vi "CreateCurveNames.vi"(0 "Exp.lvclass In":refnum<class "Experiment.lvclass">, 5 "IndCourbe":i64 caption="Numéro de Balayage", 7 "SinglePar":bool, 9 "NomDon":string[](array[string])=["RTêta;", "X&Y;"], 11 "error in":errorcluster, 12 "ScanFunc":i32) -> (2 "MultiScan":bool, 3 "ScanTableSize":i32[](array[numeric]), 4 "Experiment.lvclass Out":refnum<class "Experiment.lvclass">, 6 "Scan list":string[](array[string]), 10 "VarPar list":string[](array[string]), 13 "CalcQIndex":cluster{"Tableau":i32[]}[](array[cluster]), 14 "DataQIndex":cluster{"Tableau":i32[]}[](array[cluster]), 15 "error out":errorcluster)   [LabVIEW 2019, in "Experiment.lvclass"]
doc: "Ce Vi créer la ligne d'entête du fichier texte de sauvegarde à partir du nombre de courbe voulu."
uses:
  Experiment.lvclass
  Experiment.lvclass/Experiment.ctl
  Calculations Class/Calculations.lvclass
  Calculations Class/Calculations.lvclass/Calculations.ctl
  Calculations Class/Accessor/GetCalcEveryScanPar.vi
  DevicesClass/BaseDevice/BaseDevice.lvclass
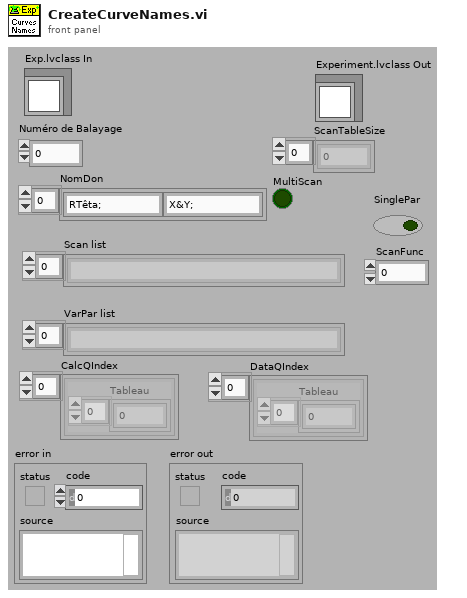
[diagram p1: front panel]
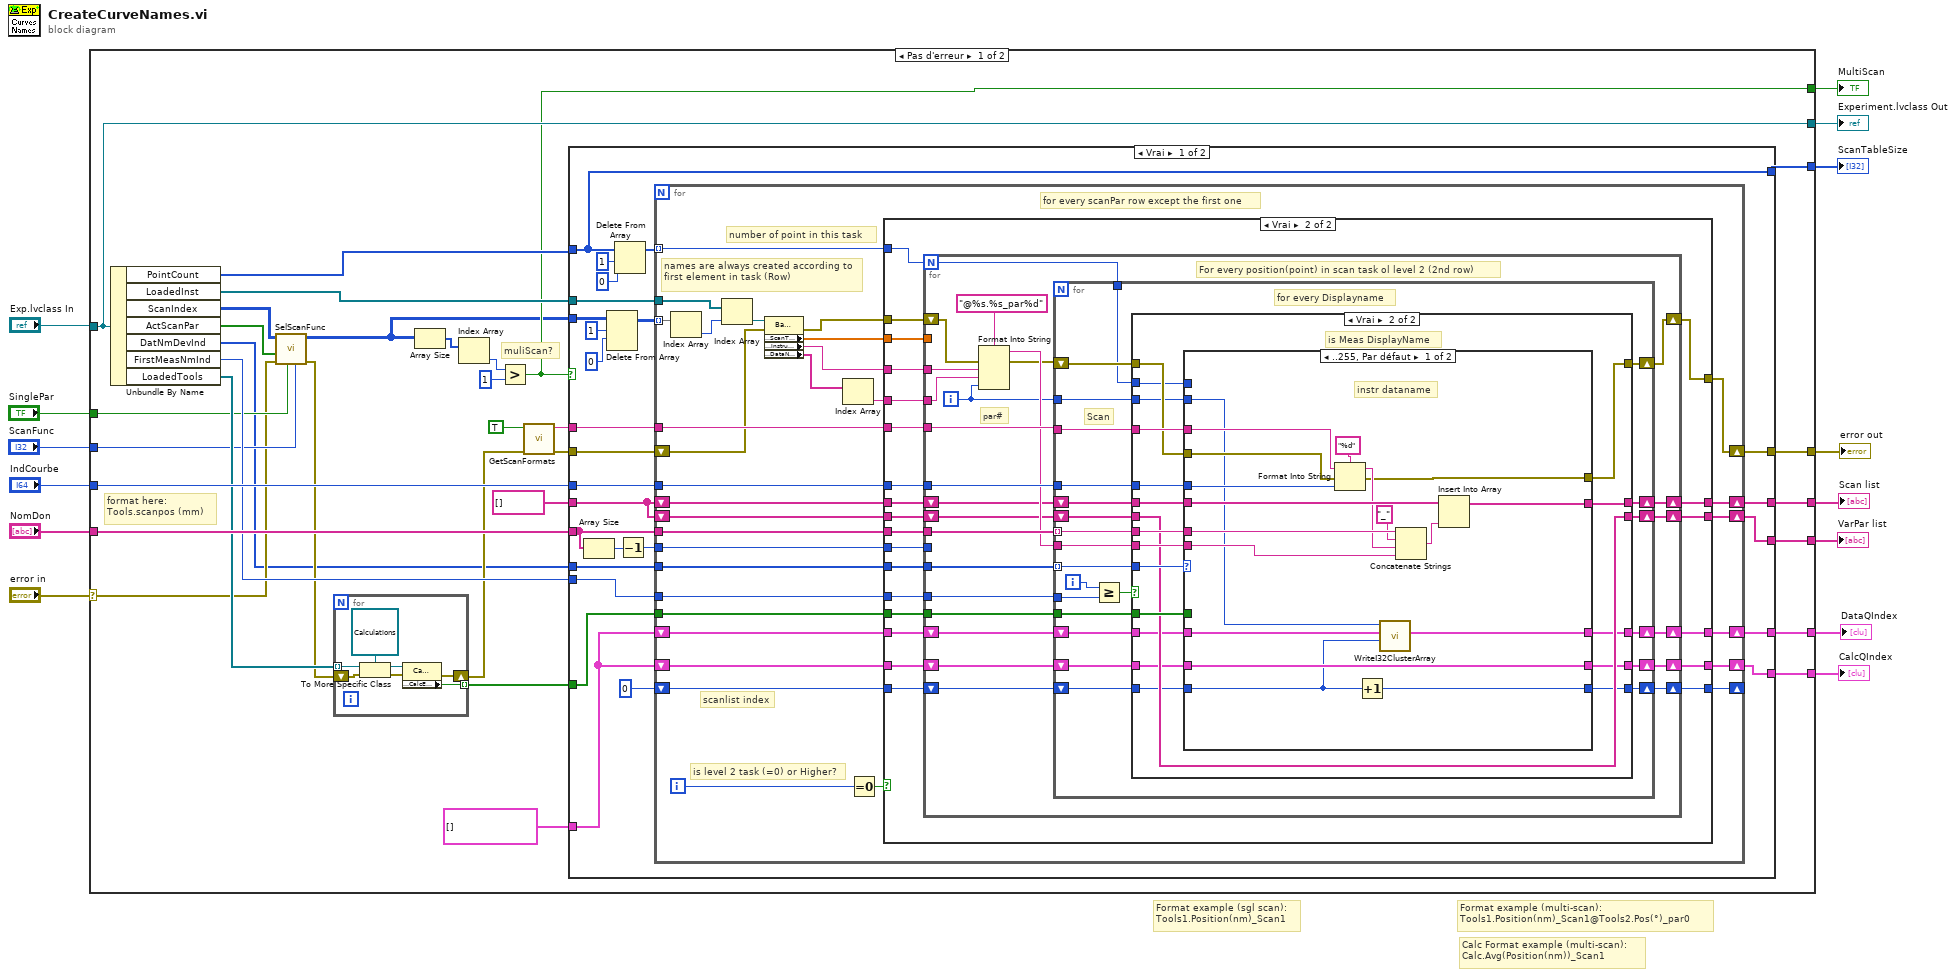
[diagram p0: block diagram]
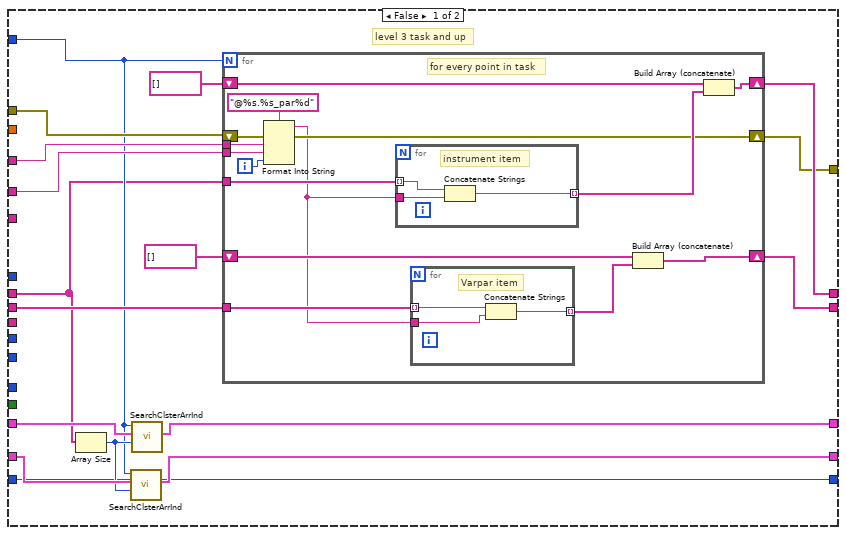
[diagram p2: hidden frame]
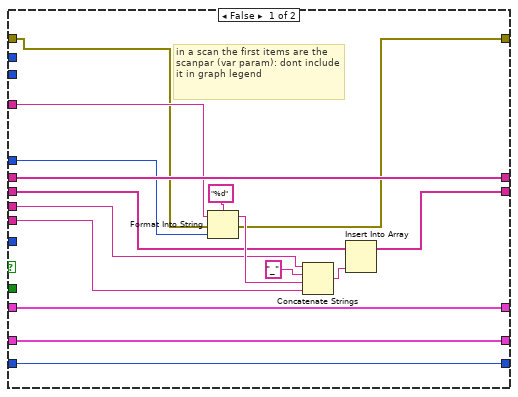
[diagram p3: hidden frame]
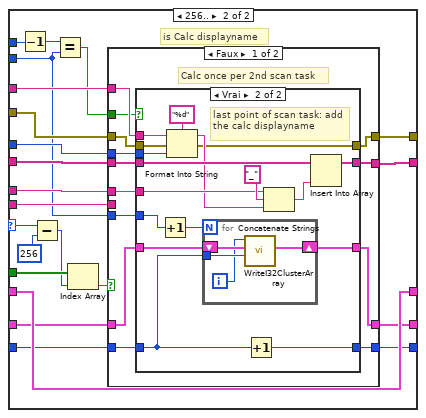
[diagram p4: hidden frame]
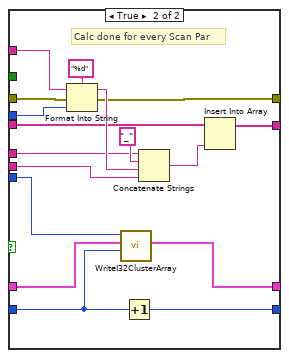
[diagram p6: hidden frame]
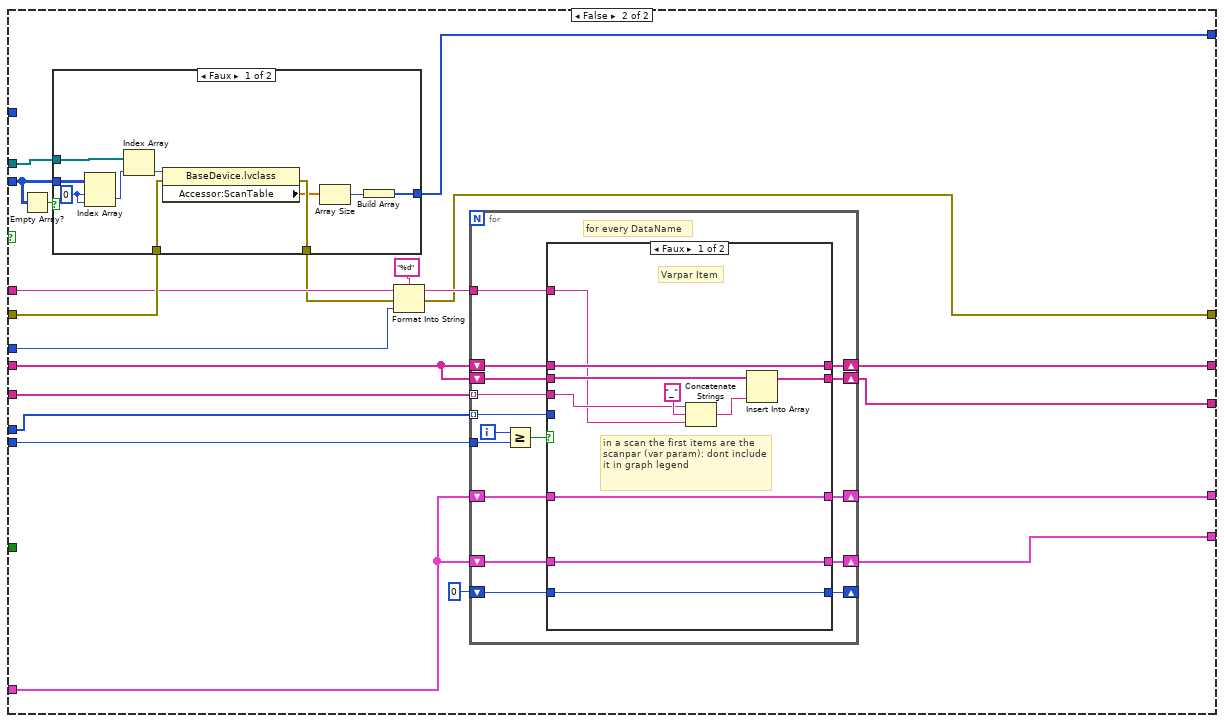
[diagram p7: hidden frame]
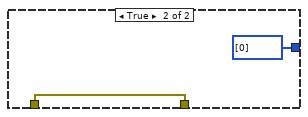
[diagram p8: hidden frame]
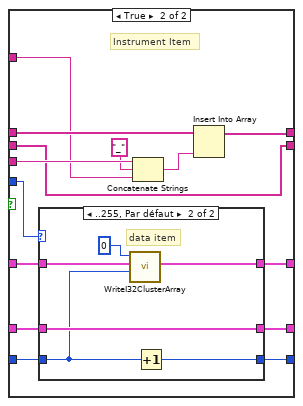
[diagram p9: hidden frame]
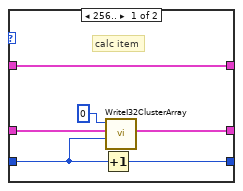
[diagram p10: hidden frame]
diagram:
  # "Calc Format example (multi-scan):\nCalc.Avg(Position(nm))_Scan1"
  # "Format example (multi-scan):\nTools1.Position(nm)_Scan1@Tools2.Pos(°)_par0"
  # "Format example (sgl scan):\nTools1.Position(nm)_Scan1"
  n1 = case shown="Pas d'erreur" "error in" {
    selector: "error in" -> [w18 w436]
    tunnel: [w38 w436] -> w13
    tunnel: [w42 _] -> w12
    tunnel: "NomDon" -> [w43 _]
    tunnel: "Exp.lvclass In" -> [w29 w435]
    tunnel: "IndCourbe" -> [w45 _]
    tunnel: [w29 w435] -> w8
    tunnel: [w36 _] -> w7
    tunnel: [w28 _] -> w6
    tunnel: [w26 _] -> w5
    tunnel: [w25 _] -> w4
    tunnel: "SinglePar" -> [w20 _]
    tunnel: "ScanFunc" -> [w19 _]
    tunnel: [w23 _] -> w1
    frame No Error {
      # "format here:\nTools.scanpos (mm)"
      # "muliScan?"
      n2 = Unbundle By Name(w29) -> ("PointCount"=w33:i32[], "LoadedInst"=w39:refnum<class "BaseDevice.lvclass">[], "ScanIndex"=w22:i32[][], "ActScanPar"=w15:bool[], "DatNmDevInd"=w16:i32[], "FirstMeasNmInd"=w37:i32, "LoadedTools"=w32:refnum<class "BaseDevice.lvclass">[])
      n3 = call "SelScanFunc.vi"("Function"=w19, "SInglePar"=w20, "ErrorIn(No Error)"=w18, "Active ScanPar"=w15, "ScanIndexIn"=w22) -> ("sortie d'erreur"=w17:errorcluster, "ScanIndexOut"=w21:i32[][])  [unwired: 4 in, 1 out]
      n4 = for {
        tunnel: w32 -> [w50] mode=indexing
        shift-right: [w48] -> w31
        shift-left: w17 -> [w49]
        tunnel: [w47] -> w30 mode=indexing
        n5 = To More Specific Class(target class=refnum<class "Calculations.lvclass"> refnum ("Calculations.lvclass"), reference=w50, error in=w49) -> (specific class reference=w52:refnum<class "Calculations.lvclass">, error out=w53:errorcluster)
        n6 = property class="Calculations.lvclass"(reference=w52, error in=w53) -> (error out=w48:errorcluster, "Accessor:CalcEveryScanPar"=w47:bool)  [unwired: 1 out]
      }
      n7 = Array Size(array=w21) -> (size(s)=w35:i32[])
      n8 = Index Array(array=w35) -> (element=w34:i32)  [unwired: 1 in]
      n9 = Greater?(x=w34, y=1) -> (0:w23:bool)
      n10 = call "GetScanFormats.vi"("ErrorIn(No Error)"=w31, "Scan(T)"=TRUE) -> ("sortie d'erreur"=w44:errorcluster, "Prefixe"=w46:string)  [unwired: 7 in, 1 out]
      n11 = case shown="Vrai" w23 {
        tunnel: w46 -> [w79 w360]
        tunnel: w45 -> [w78 w361]
        tunnel: w44 -> [w77 w365]
        tunnel: w43 -> [w64 w370]
        tunnel: [w72 w369] -> w42
        tunnel: string[] [] -> [w59 w364]
        tunnel: w21 -> [w76 w351]
        tunnel: w39 -> [w75 w367]
        tunnel: [w74 w353] -> w38
        tunnel: w37 -> [w73 w368]
        tunnel: [w60 w366] -> w36
        tunnel: w33 -> [w60 _]
        tunnel: w16 -> [w65 w357]
        tunnel: w30 -> [w61 _]
        tunnel: [w58 w363] -> w28
        tunnel: cluster{"Tableau":i32[]}[] [] ("CalcQIndex") -> [w56 w355]
        tunnel: [w55 w354] -> w26
        tunnel: [w54 w356] -> w25
        frame True {
          n12 = Array Size(array=w64) -> (size(s)=w63:i32)
          n13 = Delete From Array(array=w76, length=1 ("longueur"), index (row)=0 ("indice (ligne)")) -> (array with subset deleted=w71:i32[][])  [unwired: 1 in, 1 out]
          n14 = Delete From Array(array=w60, length=1 ("longueur"), index=0 ("indice")) -> (array with subset deleted=w67:i32[])  [unwired: 1 out]
          n15 = Decrement(x=w63) -> (x-1=w62:i32)
          n16 = for {
            tunnel: w79 -> [w110]
            tunnel: w78 -> [w109]
            tunnel: w64 -> [w108]
            tunnel: w71 -> [w107] mode=indexing
            tunnel: w75 -> [w106]
            shift-right: [w104] -> w74
            shift-left: w77 -> [w105]
            tunnel: w73 -> [w103]
            shift-right: [w100] -> w72
            shift-left: w59 -> [w99]
            tunnel: w67 -> [w80] mode=indexing
            tunnel: w65 -> [w92]
            tunnel: w61 -> [w91]
            tunnel: w62 -> [w90]
            shift-right: [w87] -> w58
            shift-left: w59 -> [w88]
            shift-right: [w85] -> _
            shift-left: 0 ("Numérique") -> [w86]
            shift-right: [w81] -> w55
            shift-left: w56 -> [w82]
            shift-right: [w83] -> w54
            shift-left: w56 -> [w84]
            i -> [w89]
            # "scanlist index"
            # "is level 2 task (=0) or Higher?"
            # "number of point in this task"
            # "names are always created according to first element in task (Row)"
            # "for every scanPar row except the first one"
            n17 = Index Array(array=w107) -> (element=w97:i32)  [unwired: 1 in]
            n18 = Index Array(array=w106, index=w97) -> (element=w96:refnum<class "BaseDevice.lvclass">)
            n19 = property class="BaseDevice.lvclass"(reference=w96, error in=w105) -> (error out=w98:errorcluster, "Accessor:ScanTable"=w94:dbl[], "Accessor:InstrumentName"=w101:string, "Accessor:DataNames"=w95:string[])  [unwired: 1 out]
            n20 = Index Array(array=w95) -> (element=w102:string)  [unwired: 1 in]
            n21 = Equal To 0?(x=w89) -> (x = 0?=w93:bool)
            n22 = case shown="Vrai" w93 {
              tunnel: w110 -> [_ w171]
              tunnel: w109 -> [_ w170]
              tunnel: w108 -> [_ w169]
              tunnel: [w125 w168] -> w104
              tunnel: w103 -> [_ w167]
              tunnel: w102 -> [w124 w166]
              tunnel: w101 -> [w123 w165]
              tunnel: [w126 w164] -> w100
              tunnel: w99 -> [w111 w163]
              tunnel: w80 -> [w112 w149]
              tunnel: w98 -> [w127 w162]
              tunnel: w94 -> [_ w161]
              tunnel: w92 -> [_ w160]
              tunnel: w91 -> [_ w159]
              tunnel: w90 -> [_ w158]
              tunnel: w88 -> [w119 w157]
              tunnel: [w122 w156] -> w87
              tunnel: w86 -> [w113 w155]
              tunnel: [w113 w154] -> w85
              tunnel: w84 -> [w118 w153]
              tunnel: [w115 w152] -> w83
              tunnel: w82 -> [w117 w151]
              tunnel: [w114 w150] -> w81
              frame False {
                # "level 3 task and up"
                n23 = Array Size(array=w111) -> (size(s)=w116:i32)
                n24 = call "SearchClsterArrInd.vi"("ScanlistSize"=w116, "array"=w117, "Currtaskparcnt"=w112) -> ("output array"=w114:cluster{"Tableau":i32[]}[])  [unwired: 7 in, 1 out]
                n25 = call "SearchClsterArrInd.vi"("ScanlistSize"=w116, "array"=w118, "Currtaskparcnt"=w112) -> ("output array"=w115:cluster{"Tableau":i32[]}[])  [unwired: 7 in, 1 out]
                n26 = for {
                  N: w112 -> [_]
                  tunnel: w123 -> [w142]
                  tunnel: w124 -> [w141]
                  shift-right: [w137] -> w125
                  shift-left: w127 -> [w140]
                  tunnel: w111 -> [w139]
                  shift-right: [w136] -> w126
                  shift-left: string[] [] -> [w135]
                  shift-right: [w133] -> w122
                  shift-left: string[] [] -> [w132]
                  tunnel: w119 -> [w131]
                  i -> [w128]
                  # "for every point in task"
                  n27 = Format Into String(format string="@%s.%s_par%d" ("chaîne de format"), error in=w140, w142, w141, w128) -> (resulting string=w129:string, error out=w137:errorcluster)  [unwired: 1 in]
                  n28 = for {
                    tunnel: w139 -> [w143] mode=indexing
                    tunnel: [w145] -> w138 mode=indexing
                    tunnel: w129 -> [w144]
                    # "instrument item"
                    n29 = Concatenate Strings(w143, w144) -> (w145:string)
                  }
                  n30 = for {
                    tunnel: w131 -> [w148] mode=indexing
                    tunnel: [w147] -> w134 mode=indexing
                    tunnel: w129 -> [w146]
                    # "Varpar item"
                    n31 = Concatenate Strings(w148, w146) -> (w147:string)
                  }
                  n32 = Build Array (concatenate)(w132, w134) -> (w133:string[])
                  n33 = Build Array (concatenate)(w135, w138) -> (w136:string[])
                }
              }
              frame True {
                n34 = for {
                  N: w149 -> [w183]
                  tunnel: w171 -> [w196]
                  tunnel: w170 -> [w195]
                  tunnel: w169 -> [w194]
                  shift-right: [w180] -> w168
                  shift-left: w162 -> [w192]
                  tunnel: w167 -> [w193]
                  tunnel: w166 -> [w191]
                  tunnel: w165 -> [w190]
                  shift-right: [w181] -> w164
                  shift-left: w163 -> [w188]
                  tunnel: w161 -> [_]
                  tunnel: w160 -> [w185]
                  tunnel: w159 -> [w184]
                  tunnel: w158 -> [_]
                  shift-right: [w178] -> w156
                  shift-left: w157 -> [w179]
                  shift-right: [w176] -> w154
                  shift-left: w155 -> [w177]
                  shift-right: [w174] -> w152
                  shift-left: w153 -> [w175]
                  shift-right: [w172] -> w150
                  shift-left: w151 -> [w173]
                  i -> [w182]
                  # "par#"
                  # "For every position(point) in scan task ol level 2 (2nd row)"
                  n35 = Format Into String(format string="@%s.%s_par%d" ("chaîne de format"), error in=w192, w190, w191, w182) -> (resulting string=w189:string, error out=w187:errorcluster)  [unwired: 1 in]
                  n36 = for {
                    tunnel: w196 -> [w214]
                    tunnel: w194 -> [w217] mode=indexing
                    shift-right: [w218] -> w181
                    shift-left: w188 -> [w219]
                    tunnel: w195 -> [w215]
                    shift-right: [w205] -> w180
                    shift-left: w187 -> [w213]
                    tunnel: w193 -> [w212]
                    tunnel: w189 -> [w211]
                    tunnel: w185 -> [w210] mode=indexing
                    tunnel: w184 -> [w209]
                    tunnel: w183 -> [w207]
                    tunnel: w182 -> [w206]
                    shift-right: [w203] -> w178
                    shift-left: w179 -> [w204]
                    shift-right: [w201] -> w176
                    shift-left: w177 -> [w202]
                    shift-right: [w199] -> w174
                    shift-left: w175 -> [w200]
                    shift-right: [w197] -> w172
                    shift-left: w173 -> [w198]
                    i -> [w208]
                    # "Scan"
                    # "for every Displayname"
                    n37 = Greater Or Equal?(x=w208, y=w212) -> (x >= y?=w216:bool)
                    n38 = case shown="Vrai" w216 {
                      tunnel: w219 -> [w235 w254]
                      tunnel: [w235 w253] -> w218
                      tunnel: w217 -> [w229 w252]
                      tunnel: w215 -> [w223 w248]
                      tunnel: w214 -> [w230 w251]
                      tunnel: w213 -> [w227 w250]
                      tunnel: w211 -> [w228 w249]
                      tunnel: w210 -> [_ w246]
                      tunnel: w209 -> [_ w247]
                      tunnel: w207 -> [_ w245]
                      tunnel: w206 -> [_ w244]
                      tunnel: [w226 w243] -> w205
                      tunnel: w204 -> [w225 w242]
                      tunnel: [w224 w242] -> w203
                      tunnel: w202 -> [w222 w237]
                      tunnel: [w222 w236] -> w201
                      tunnel: w200 -> [w221 w241]
                      tunnel: [w221 w240] -> w199
                      tunnel: w198 -> [w220 w239]
                      tunnel: [w220 w238] -> w197
                      frame False {
                        # "in a scan the first items are the scanpar (var param): dont include it in graph legend"
                        n39 = Format Into String(format string="%d" ("chaîne de format"), initial string=w230, error in=w227, w223) -> (resulting string=w233:string, error out=w226:errorcluster)
                        n40 = Concatenate Strings(w229, "_" ("chaîne"), w233, w228) -> (w234:string)
                        n41 = Insert Into Array(array=w225, new element=w234) -> (w224:string[])  [unwired: 1 in]
                      }
                      frame True {
                        # "is Meas DisplayName"
                        n42 = case shown="..255, Par défaut" w246 {
                          selector: w246 -> [_ w285]
                          tunnel: w254 -> [w272 w291]
                          tunnel: [w271 w289] -> w253
                          tunnel: w252 -> [w270 w292]
                          tunnel: w251 -> [w269 w294]
                          tunnel: w250 -> [w268 w280]
                          tunnel: w249 -> [w264 w290]
                          tunnel: w248 -> [w263 w293]
                          tunnel: w247 -> [_ w288]
                          tunnel: w245 -> [_ w284]
                          tunnel: w244 -> [w258 w276]
                          tunnel: [w261 w281] -> w243
                          tunnel: w241 -> [w260 w278]
                          tunnel: w237 -> [w256 w273]
                          tunnel: [w259 w278] -> w240
                          tunnel: w239 -> [w257 w277]
                          tunnel: [w257 w275] -> w238
                          tunnel: [w255 w274] -> w236
                          frame ..255, Default {
                            # "instr dataname"
                            n43 = Format Into String(format string="%d" ("chaîne de format"), initial string=w269, error in=w268, w263) -> (resulting string=w266:string, error out=w261:errorcluster)
                            n44 = Increment(x=w256) -> (x+1=w255:i32)
                            n45 = call <userlib>:"WriteI32ClusterArray.vi"("Data"=w256, "array"=w260, "ClusterInd"=w258) -> ("output array"=w259:cluster{"Tableau":i32[]}[])  [unwired: 7 in, 1 out]
                            n46 = Concatenate Strings(w270, "_" ("chaîne"), w266, w264) -> (w267:string)
                            n47 = Insert Into Array(array=w272, new element=w267) -> (w271:string[])  [unwired: 1 in]
                          }
                          frame 256.. {
                            # "is Calc displayname"
                            n48 = Decrement(x=w284) -> (x-1=w283:i32)
                            n49 = Subtract(x=w285, y=256) -> (x-y=w287:i32)
                            n50 = Equal?(x=w283, y=w276) -> (x = y?=w282:bool)
                            n51 = Index Array(array=w288, index=w287) -> (element=w279:bool)
                            n52 = case shown="Faux" w279 {
                              tunnel: w294 -> [w303 w345]
                              tunnel: w293 -> [w307 w344]
                              tunnel: w292 -> [w305 w343]
                              tunnel: w291 -> [w306 w342]
                              tunnel: w290 -> [_ w340]
                              tunnel: [w304 w341] -> w289
                              tunnel: w282 -> [w302 _]
                              tunnel: [w301 w339] -> w281
                              tunnel: w280 -> [w300 w338]
                              tunnel: w277 -> [w299 w335]
                              tunnel: w273 -> [w296 w334]
                              tunnel: w276 -> [w297 w337]
                              tunnel: [w298 w336] -> w275
                              tunnel: [w295 w333] -> w274
                              frame False {
                                # "Calc once per 2nd scan task"
                                n53 = case shown="Vrai" w302 {
                                tunnel: w303 -> [_ w327]
                                tunnel: w307 -> [_ w326]
                                tunnel: w306 -> [w311 w323]
                                tunnel: w305 -> [_ w322]
                                tunnel: [w311 w320] -> w304
                                tunnel: [w310 w319] -> w301
                                tunnel: w300 -> [w310 w318]
                                tunnel: w299 -> [w309 w314]
                                tunnel: [w309 w316] -> w298
                                tunnel: w297 -> [_ w317]
                                tunnel: w296 -> [w308 w315]
                                tunnel: [w308 w313] -> w295
                                frame False {
                                }
                                frame True {
                                # "last point of scan task: add the calc displayname"
                                n54 = Increment(x=w317) -> (x+1=w312:i32)
                                n55 = Format Into String(format string="%d" ("chaîne de format"), initial string=w327, error in=w318, w326) -> (resulting string=w321:string, error out=w319:errorcluster)
                                n56 = for {
                                N: w312 -> [_]
                                tunnel: w315 -> [w331]
                                shift-right: [w329] -> w316
                                shift-left: w314 -> [w332]
                                i -> [w330]
                                n57 = call <userlib>:"WriteI32ClusterArray.vi"("Data"=w331, "array"=w332, "ClusterInd"=w330) -> ("output array"=w329:cluster{"Tableau":i32[]}[])  [unwired: 7 in, 1 out]
                                }
                                n58 = Increment(x=w315) -> (x+1=w313:i32)
                                n59 = Concatenate Strings(w322, "_" ("chaîne"), w321) -> (w324:string)
                                n60 = Insert Into Array(array=w323, new element=w324) -> (w320:string[])  [unwired: 1 in]
                                }
                                }
                              }
                              frame True {
                                # "Calc done for every Scan Par"
                                n61 = Format Into String(format string="%d" ("chaîne de format"), initial string=w345, error in=w338, w344) -> (resulting string=w347:string, error out=w339:errorcluster)
                                n62 = call <userlib>:"WriteI32ClusterArray.vi"("Data"=w334, "array"=w335, "ClusterInd"=w337) -> ("output array"=w336:cluster{"Tableau":i32[]}[])  [unwired: 7 in, 1 out]
                                n63 = Increment(x=w334) -> (x+1=w333:i32)
                                n64 = Concatenate Strings(w343, "_" ("chaîne"), w347, w340) -> (w346:string)
                                n65 = Insert Into Array(array=w342, new element=w346) -> (w341:string[])  [unwired: 1 in]
                              }
                            }
                          }
                        }
                      }
                    }
                  }
                }
              }
            }
          }
        }
        frame False {
          n66 = Empty Array?(array=w351) -> (empty?=w350:bool)
          n67 = case shown="Faux" w350 {
            tunnel: w351 -> [w380 _]
            tunnel: w367 -> [w379 _]
            tunnel: [w378 i32[] [0]] -> w366
            tunnel: w365 -> [w377 w382]
            tunnel: [w376 w382] -> w358
            frame False {
              w373 = 0 ("indice (ligne)")
              n68 = Index Array(array=w380, index (row)=w373, index (col)=w373) -> (element=w375:i32)
              n69 = Index Array(array=w379, index=w375) -> (element=w374:refnum<class "BaseDevice.lvclass">)
              n70 = property class="BaseDevice.lvclass"(reference=w374, error in=w377) -> (error out=w376:errorcluster, "Accessor:ScanTable"=w372:dbl[])  [unwired: 1 out]
              n71 = Array Size(array=w372) -> (size(s)=w371:i32)
              n72 = Build Array(w371) -> (w378:i32[])
            }
            frame True {
            }
          }
          n73 = Format Into String(format string="%d" ("chaîne de format"), initial string=w360, error in=w358, w361) -> (resulting string=w359:string, error out=w353:errorcluster)
          n74 = for {
            tunnel: w359 -> [w394]
            tunnel: w370 -> [w396] mode=indexing
            shift-right: [w397] -> w369
            shift-left: w364 -> [w398]
            tunnel: w368 -> [w393]
            shift-right: [w391] -> w363
            shift-left: w364 -> [w392]
            tunnel: w357 -> [w390] mode=indexing
            shift-right: [w386] -> w356
            shift-left: w355 -> [w385]
            shift-right: [w388] -> w354
            shift-left: w355 -> [w389]
            shift-right: [w383] -> _
            shift-left: 0 ("Data") -> [w384]
            i -> [w387]
            # "for every DataName"
            n75 = Greater Or Equal?(x=w387, y=w393) -> (x >= y?=w395:bool)
            n76 = case shown="Faux" w395 {
              tunnel: w398 -> [w408 w422]
              tunnel: [w408 w421] -> w397
              tunnel: w396 -> [w403 w420]
              tunnel: w394 -> [w402 w418]
              tunnel: w392 -> [w405 w419]
              tunnel: [w404 w419] -> w391
              tunnel: w390 -> [_ w415]
              tunnel: w389 -> [w401 w414]
              tunnel: [w401 w413] -> w388
              tunnel: w384 -> [w399 w412]
              tunnel: [w400 w411] -> w386
              tunnel: w385 -> [w400 w410]
              tunnel: [w399 w409] -> w383
              frame False {
                # "in a scan the first items are the scanpar (var param): dont include it in graph legend"
                # "Varpar Item"
                n77 = Concatenate Strings(w403, "_" ("chaîne"), w402) -> (w407:string)
                n78 = Insert Into Array(array=w405, new element=w407) -> (w404:string[])  [unwired: 1 in]
              }
              frame True {
                # "Instrument Item"
                n79 = case shown="..255, Par défaut" w415 {
                  tunnel: w414 -> [w428 w434]
                  tunnel: [w427 w434] -> w413
                  tunnel: w412 -> [w424 w430]
                  tunnel: [w425 w431] -> w411
                  tunnel: w410 -> [w425 w432]
                  tunnel: [w423 w429] -> w409
                  frame 256.. {
                    # "calc item"
                    n80 = Increment(x=w424) -> (x+1=w423:i32)
                    n81 = call <userlib>:"WriteI32ClusterArray.vi"("Data"=w424, "array"=w428, "ClusterInd"=0) -> ("output array"=w427:cluster{"Tableau":i32[]}[])  [unwired: 7 in, 1 out]
                  }
                  frame ..255, Default {
                    # "data item"
                    n82 = call <userlib>:"WriteI32ClusterArray.vi"("Data"=w430, "array"=w432, "ClusterInd"=0) -> ("output array"=w431:cluster{"Tableau":i32[]}[])  [unwired: 7 in, 1 out]
                    n83 = Increment(x=w430) -> (x+1=w429:i32)
                  }
                }
                n84 = Concatenate Strings(w420, "_" ("chaîne"), w418) -> (w417:string)
                n85 = Insert Into Array(array=w422, new element=w417) -> (w421:string[])  [unwired: 1 in]
              }
            }
          }
        }
      }
    }
    frame Error {
    }
  }
  "error out" <- w13
  "Scan list" <- w12
  "Experiment.lvclass Out" <- w8
  "ScanTableSize" <- w7
  "VarPar list" <- w6
  "CalcQIndex" <- w5
  "DataQIndex" <- w4
  "MultiScan" <- w1
